vi "Module Loop.vi"(8 "error in (no error)":errorcluster, 11 "TestModule in":refnum<class "TestModule.lvclass">) -> (0 "error out":errorcluster, 3 "TestModule out":refnum<class "TestModule.lvclass">)   [LabVIEW 2020, in "VolatusScratch.lvlib" / "TestModule.lvclass"]
uses:
  TestModule.lvclass
  C:/dev/lv20CE/relink/lv-volatus/Volatus/Module/Module.lvclass
  Volatus/Module/Module.lvclass/Module.ctl
  Volatus/MessageQ/MessageQ.lvclass/MessageQ.ctl
  Volatus/Module/Module.lvclass
  TestModule.lvclass/TestModule.ctl
  Volatus/VolatusAPI/VolatusAPI.lvclass/VolatusAPI.ctl
  messages/TwoDoubles/Class/Msg.lvclass
  C:/dev/lv20CE/relink/lv-protoc/LV-Proto/Message/Message.lvclass
  messages/TwoDoubles/Class/Msg.lvclass/Msg.ctl
  messages/Double/Class/Msg.lvclass/Msg.ctl
  lv-vecto/Vecto/Group DBL/Group DBL.lvclass
  C:/dev/lv20CE/relink/lv-vecto/Vecto/Group/Group.lvclass
  messages/Double/Class/Msg.lvclass
  lv-vecto/Vecto/TCPMessageService/Reply.vi
  <vilib>/Utility/error.llb/Error Cluster From Error Code.vi
  lv-protoc/LV-Proto/Message/Message.lvclass
  Volatus/MessageQ/MessageQ.lvclass
  Volatus/Volatus.lvlib
  Volatus/VolatusAPI/VolatusAPI.lvclass
panel:
  out "LED":bool
  in  "Values":dbl[](array[slide])=[0.0, 0.0, 0.0, 0.0, 0.0] scale=0.0..10.0
  out "i":i32
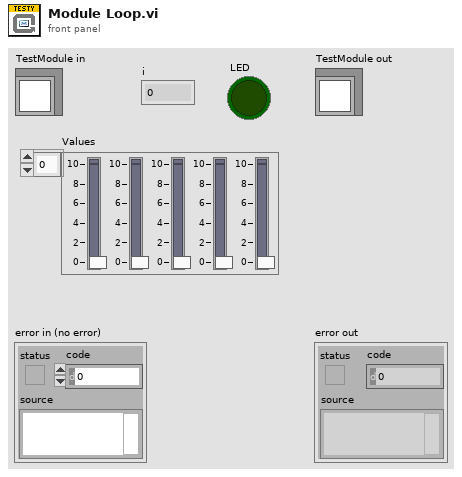
[diagram p1: front panel]
types:
  T1 = enum32{"Invalid", "Standard", "Closed", "Hidden", "Minimized", "Maximized"}
  T2 = typedef "TcpPayload.lvlib/Data.ctl" = cluster{"target_node":u32, "source_id":u32, "sequence":u32, "timestamp":i64, "type":string, "task_id":string, "payload":u8[]}
  T3 = typedef "TwoDoubles.lvlib/Data.ctl" = cluster{"a":dbl, "b":dbl}
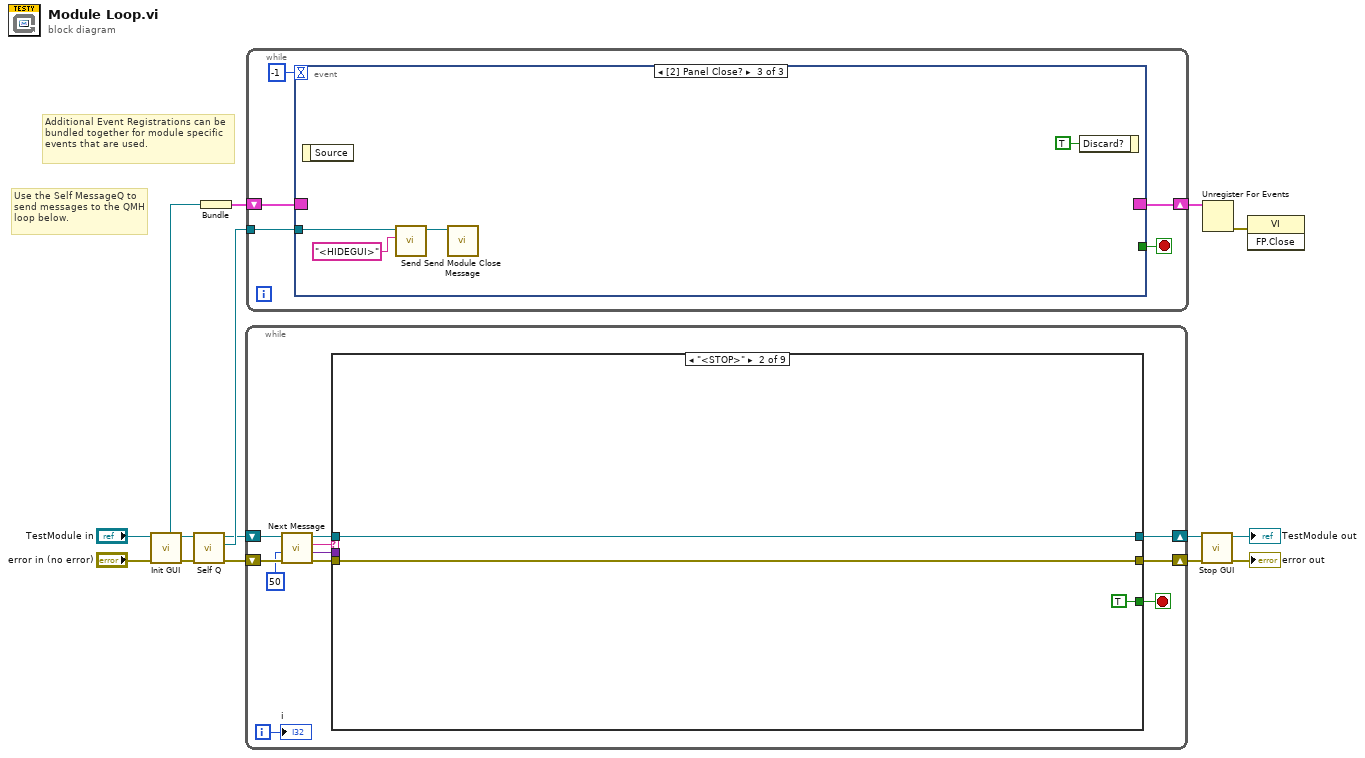
[diagram p0: block diagram]
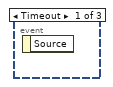
[diagram p2: hidden frame]
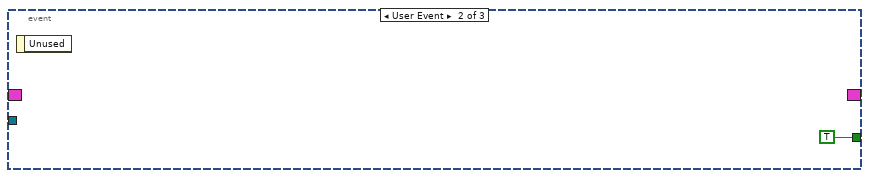
[diagram p3: hidden frame]
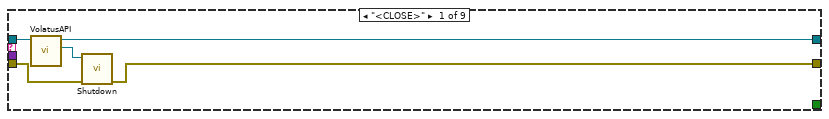
[diagram p4: hidden frame]
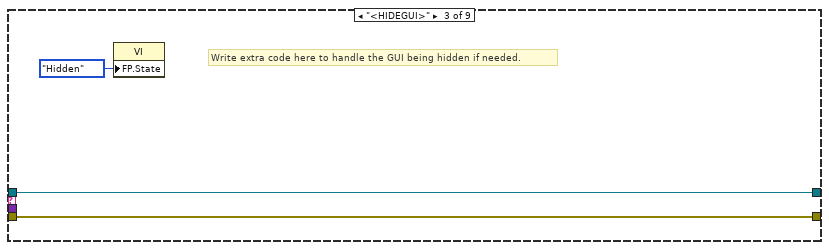
[diagram p5: hidden frame]
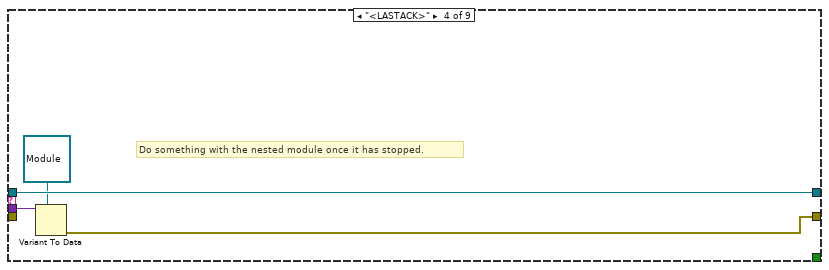
[diagram p6: hidden frame]
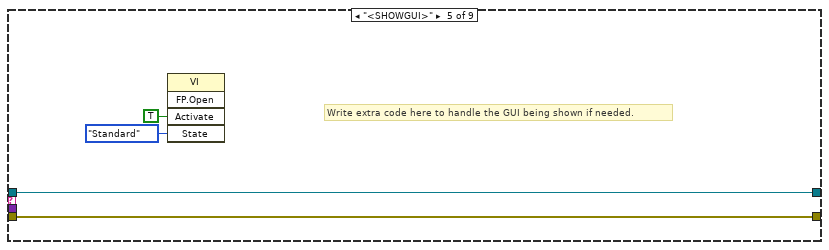
[diagram p7: hidden frame]
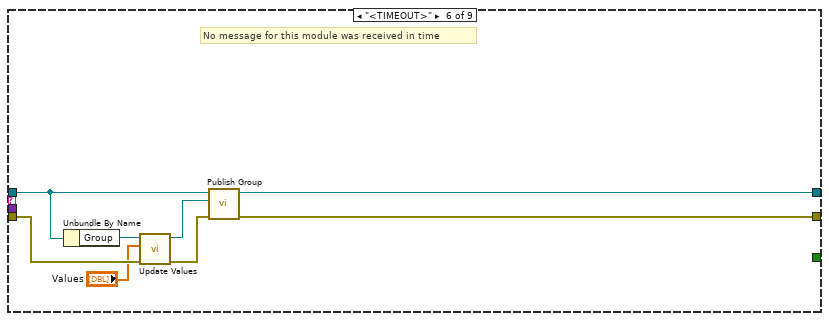
[diagram p8: hidden frame]
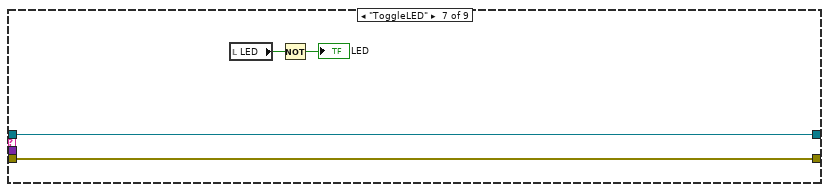
[diagram p9: hidden frame]
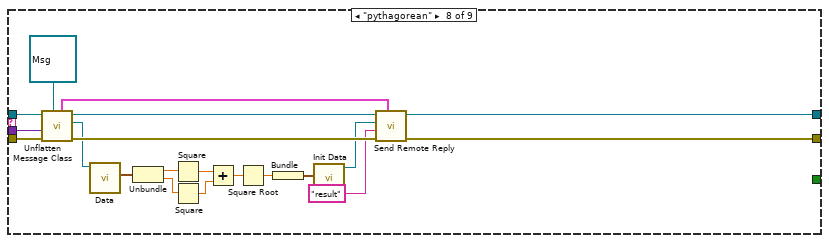
[diagram p10: hidden frame]
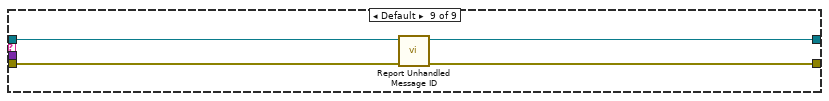
[diagram p11: hidden frame]
diagram:
  # "Additional Event Registrations can be bundled together for module specific events that are used."
  # "Use the Self MessageQ to send messages to the QMH loop below."
  n1 = call "Init GUI.vi"("Module in"="TestModule in") -> ("Module out"=w7:refnum<class "TestModule.lvclass">, "Event Reg"=w12:refnum<event-registration>)  [unwired: 9 in]
  n2 = call "Self Q.vi"("Module in"=w7) -> ("Self Q"=w6:refnum<class "MessageQ.lvclass">, "Module out"=w5:refnum<class "TestModule.lvclass">)  [unwired: 9 in]
  n3 = Bundle("Event Reg"=w12) -> (w8:cluster{"Event Reg":refnum<event-registration>})  [unwired: 1 in]
  n4 = while {
    shift-right: [w19] -> w10
    shift-left: w5 -> [w24]
    shift-right: [w18] -> w11
    shift-left: "error in (no error)" -> [w23]
    i -> [w15]
    stop <- w17 stop-if-true
    n5 = call "Next Message.vi"("error in (no error)"=w23, "Timeout ms (-1)"=50, "Module in"=w24) -> ("error out"=w22:errorcluster, "Data"=w16:variant, "ID"=w21:string, "Module out"=w20:refnum<class "TestModule.lvclass">)  [unwired: 5 in]
    n6 = case shown="\"<STOP>\"" w21 {
      tunnel: w22 -> [w26 w31 w34 _ w42 w51 w54 w75 w79]
      tunnel: w20 -> [w29 w32 w35 w39 w43 w46 w55 w73 w77]
      tunnel: [w28 w32 w35 w39 w43 w47 w55 w59 w76] -> w19
      tunnel: [w25 w31 w34 w36 w42 w48 w54 w61 w78] -> w18
      tunnel: [_ TRUE _ _ _ _ _ _ _] -> w17
      tunnel: w16 -> [_ _ _ w38 _ _ _ w72 _]
      frame "<CLOSE>" {
        n7 = call "VolatusAPI.vi"("Module in"=w29) -> ("VolatusAPI"=w27:refnum<class "VolatusAPI.lvclass">, "Module out"=w28:refnum<class "TestModule.lvclass">)  [unwired: 9 in]
        n8 = call "Shutdown.vi"("error in (no error)"=w26, "VolatusAPI in"=w27) -> ("error out"=w25:errorcluster)  [unwired: 8 in, 1 out]
      }
      frame "<STOP>" {
      }
      frame "<HIDEGUI>" {
        # "Write extra code here to handle the GUI being hidden if needed."
        n9 = property class="VI"("FP.State"=T1."Hidden" ("Front Panel Window:State")) -> ()  [unwired: 2 in, 2 out]
      }
      frame "<LASTACK>" {
        # "Do something with the nested module once it has stopped."
        n10 = Variant To Data(type=refnum<class "Module.lvclass"> refnum ("Volatus:Module"), Variant=w38) -> (error out=w36:errorcluster)  [unwired: 1 in, 1 out]
      }
      frame "<SHOWGUI>" {
        # "Write extra code here to handle the GUI being shown if needed."
        n11 = invoke class="VI" method="FP.Open"("Activate"=TRUE ("Activate?"), "State"=T1."Standard") -> ()  [unwired: 3 in, 5 out]
      }
      frame "<TIMEOUT>" {
        # "No message for this module was received in time"
        n12 = Unbundle By Name(w46) -> ("Group"=w50:refnum<class "Group DBL.lvclass">)
        n13 = call "Update Values.vi"("error in (no error)"=w51, "Values"="Values", "Group in"=w50) -> ("error out"=w44:errorcluster, "Group out"=w45:refnum<class "Group DBL.lvclass">)  [unwired: 7 in]
        n14 = call "Publish Group.vi"("error in (no error)"=w44, "Group"=w45, "Module in"=w46) -> ("error out"=w48:errorcluster, "Module out"=w47:refnum<class "TestModule.lvclass">)  [unwired: 7 in]
      }
      frame "ToggleLED" {
        n15 = local read "LED"() -> (w52:bool)
        n16 = Not(x=w52) -> (.not. x?=→"LED":bool)
      }
      frame "pythagorean" {
        n17 = call "Unflatten Message Class.vi"("Message Type"=refnum<class "Msg.lvclass"> refnum ("TwoDoubles.lvlib:Msg.lvclass"), "error in (no error)"=w75, "Data"=w72, "Module in"=w73) -> ("error out"=w74:errorcluster, "Message"=w70:refnum<class "Msg.lvclass">, "Module out"=w60:refnum<class "TestModule.lvclass">, "TcpPayload"=w57:T2)  [unwired: 4 in]
        n18 = call "Data.vi"("PB Msg Template in"=w70) -> ("Data"=w69:T3)  [unwired: 8 in, 2 out]
        n19 = Unbundle(w69) -> ("a"=w68:dbl, "b"=w67:dbl)
        n20 = Square(x=w68) -> (x^2=w66:dbl)
        n21 = Square(x=w67) -> (x^2=w65:dbl)
        n22 = Add(x=w66, y=w65) -> (x+y=w64:dbl)
        n23 = Square Root(x=w64) -> (sqrt(x)=w63:dbl)
        n24 = Bundle(w63) -> (w62:cluster{dbl})  [unwired: 1 in]
        n25 = call "Init Data.vi"("Data"=w62) -> ("Msg out"=w58:refnum<class "Msg.lvclass">)  [unwired: 10 in]
        n26 = call "Send Remote Reply.vi"("Original Payload"=w57, "error in (no error)"=w74, "Message Type"="result", "Message"=w58, "Module in"=w60) -> ("error out"=w61:errorcluster, "Module out"=w59:refnum<class "TestModule.lvclass">)  [unwired: 5 in]
      }
      frame Default {
        n27 = call "Report Unhandled Message ID.vi"("error in (no error)"=w79, "Module in"=w77) -> ("error out"=w78:errorcluster, "Module out"=w76:refnum<class "TestModule.lvclass">)  [unwired: 8 in]
      }
    }
    "i" <- w15
  }
  n28 = while {
    tunnel: w6 -> [w84]
    shift-right: [w82] -> w9
    shift-left: w8 -> [w83]
    stop <- w81 stop-if-true
    n29 = event shown="[2] Panel Close?" {
      selector: w83 -> [_ _ _]
      dyn-events: [_ _ _] -> w82
      timeout: -1 -> [_ _ _]
      tunnel: w84 -> [_ _ w88]
      tunnel: [_ TRUE _] -> w81
      event Timeout {
        n30 = event-data() -> ()  [unwired: 1 in, 1 out]
      }
      event User Event {
        n31 = event-data() -> ()  [unwired: 1 in, 1 out]
      }
      event Panel Close? {
        n32 = event-data() -> ()  [unwired: 1 in, 1 out]
        n33 = call "Send.vi"("ID"="<HIDEGUI>", "MessageQ in"=w88) -> ("MessageQ out"=w86:refnum<class "MessageQ.lvclass">)  [unwired: 8 in, 1 out]
        n34 = call "Send Module Close Message.vi"("MessageQ"=w86) -> ()  [unwired: 10 in, 1 out]
        n35 = event-data("Discard?"=TRUE) -> ()  [unwired: 1 in, 1 out]
      }
    }
  }
  n36 = call "Stop GUI.vi"("error in (no error)"=w11, "Module in"=w10) -> ("error out"=→"error out":errorcluster, "Module out"=→"TestModule out":refnum<class "TestModule.lvclass">)  [unwired: 8 in]
  n37 = Unregister For Events(event registration refnum=w9) -> (error out=w13:errorcluster)  [unwired: 1 in]
  n38 = invoke class="VI" method="FP.Close"(error in=w13) -> ()  [unwired: 2 in, 3 out]
